vi "LoadConfiguration.vi"(0 "instruction target in":refnum<class "niInstr Instruction Target v1 Host.lvclass">, 5 "SVPWMContext in":refnum<class "niInstr Instruction Framework Context v1 Host.lvclass">, 7 "Configuration":T1, 11 "error in (no error)":errorcluster) -> (4 "instruction target out":refnum<class "niInstr Instruction Target v1 Host.lvclass">, 6 "SVPWMContext out":refnum<class "niInstr Instruction Framework Context v1 Host.lvclass">, 15 "error out":errorcluster)   [LabVIEW 2015, in "SVPWMInterface.lvlib"]
uses:
  SVPWMInterface.lvlib
  <instrlib>/_niInstr/Instruction Framework/v1/Host/Instruction Framework Context/niInstr Instruction Framework Context v1 Host.lvclass
  <instrlib>/_niInstr/Instruction Framework/v1/Host/Instruction Target/niInstr Instruction Target v1 Host.lvclass
  Configuration.ctl
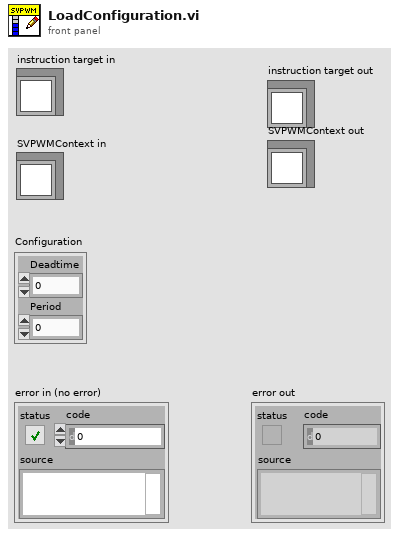
[diagram p1: front panel]
types:
  T1 = typedef "SVPWMInterface.lvlib/Configuration.ctl" = cluster{"Deadtime":u8, "Period":u32}
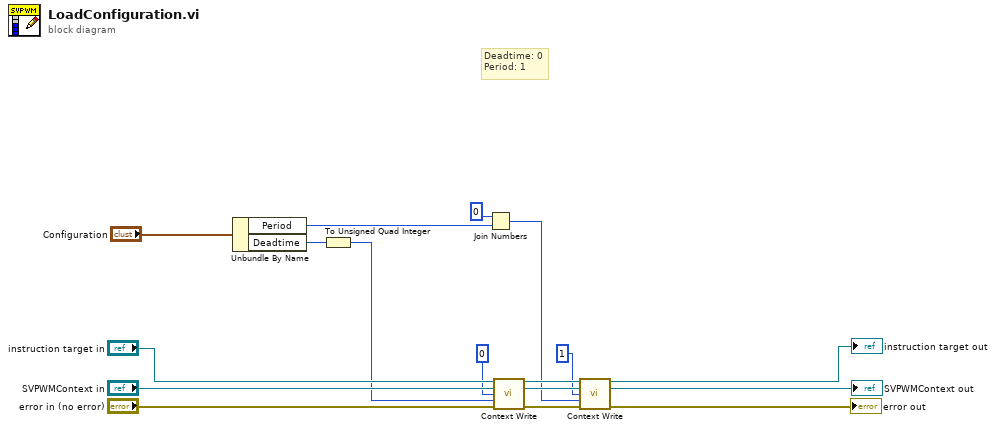
[diagram p0: block diagram]
diagram:
  # "Deadtime: 0\nPeriod: 1"
  n1 = Unbundle By Name("Configuration") -> ("Period"=w1:u32, "Deadtime"=w2:u8)
  n2 = To Unsigned Quad Integer(1:w2) -> (0:w3:u64)
  n3 = Join Numbers(hi=u32 0, lo=w1) -> ((hi.lo)=w8:u64)
  n4 = call <instrlib>:"Context Write.vi"("instruction target in"="instruction target in", "context in"="SVPWMContext in", "address"=u64 0, "data"=w3, "error in"="error in (no error)") -> ("instruction target out"=w14:refnum<class "niInstr Instruction Target v1 Host.lvclass">, "context out"=w13:refnum<class "niInstr Instruction Framework Context v1 Host.lvclass">, "error out"=w12:errorcluster)  [unwired: 8 in]
  n5 = call <instrlib>:"Context Write.vi"("instruction target in"=w14, "context in"=w13, "address"=u64 1, "data"=w8, "error in"=w12) -> ("instruction target out"=→"instruction target out":refnum<class "niInstr Instruction Target v1 Host.lvclass">, "context out"=→"SVPWMContext out":refnum<class "niInstr Instruction Framework Context v1 Host.lvclass">, "error out"=→"error out":errorcluster)  [unwired: 8 in]
